vi "canDataSort.vi"() -> ()   [LabVIEW 2023] (continued)
\n       223  0CF102A7   00000004    8        30\t75\tE0\t2E\t80\tFF\tFF\tFD\r\n       247  1FFFFFFF   00000004    8        00\t00\tFF\tFF\tFF\tFF\tFF\tFF\r\n       246  18F121F0   00000004    8        09\t16\t00\t00\tFF\tFF\tB0\t01\r\n       246  18F106A7   00000004    8        00\tF7\tFF\tFF\tFF\tFF\tFF\t75\r\n       245  0CF104A7   00000004    8        F0\t60\t22\tFC\tFF\tFF\tFF\t3A\r\n       244  0CF103A7   00000004    8        17\t1F\t08\t60\tB1\t1F\t08\t3A\r\n       244  0CF102A7   00000004    8        30\t75\tE0\t2E\t80\tFF\tFF\tFD\r\n       243  0C3C4D4A   00000004    8        BE\tFF\tFF\t7F\t18\tFF\tFF\t3A\r\n       243  0CF101A7   00000004    8        68\t00\t97\tCC\t00\t15\t39\t26\r\n       242  18F120F0   00000004    8        2B\t75\t60\tB1\tB0\t01\tFF\tFF\r\n       241  18F11FF0   00000004    8        FF\t3F\t90\t68\t88\t1B\t10\tAC\r\n       232  1FFFFFFF   00000004    8        00\t00\tFF\tFF\tFF\tFF\tFF\tFF\r\n       252  1FFFFFFF   00000004    8        00\t00\tFF\tFF\tFF\tFF\tFF\tFF\r\n       247  1FFFFFFF   00000004    8        00\t00\tFF\tFF\tFF\tFF\tFF\tFF\r\n       246  18F121F0   00000004    8        09\t16\t00\t00\tFF\tFF\tB0\t01\r\n       246  18F106A7   00000004    8        00\tF7\tFF\tFF\tFF\tFF\tFF\t75\r\n       245  0CF104A7   00000004    8        F0\t60\t22\tFC\tFF\tFF\tFF\t3A\r\n       244  0CF103A7   00000004    8        17\t1F\t08\t60\tB1\t1F\t08\t3A\r\n       244  0CF102A7   00000004    8        30\t75\tE0\t2E\t80\tFF\tFF\tFD\r\n       243  0C3C4D4A   00000004    8        BE\tFF\tFF\t7F\t18\tFF\tFF\t3A\r\n       243  0CF101A7   00000004    8        68\t00\t97\tCC\t00\t15\t39\t26\r\n       242  18F120F0   00000004    8        2B\t75\t60\tB1\tB0\t01\tFF\tFF\r\n       241  18F11FF0   00000004    8        FF\t3F\t90\t68\t88\t1B\t10\tAC\r\n       262  1FFFFFFF   00000004    8        00\t20\tFF\tFF\tFF\tFF\tFF\tFF\r\n       252  1FFFFFFF   00000004    8        00\t00\tFF\tFF\tFF\tFF\tFF\tFF\r\n       247  1FFFFFFF   00000004    8        00\t00\tFF\tFF\tFF\tFF\tFF\tFF\r\n       246  18F121F0   00000004    8        09\t16\t00\t00\tFF\tFF\tB0\t01\r\n       246  18F106A7   00000004    8        00\tF7\tFF\tFF\tFF\tFF\tFF\t75\r\n       245  0CF104A7   00000004    8        F0\t60\t22\tFC\tFF\tFF\tFF\t3A\r\n       244  0CF103A7   00000004    8        17\t1F\t08\t60\tB1\t1F\t08\t3A\r\n       244  0CF102A7   00000004    8        30\t75\tE0\t2E\t80\tFF\tFF\tFD\r\n       243  0C3C4D4A   00000004    8        BE\tFF\tFF\t7F\t18\tFF\tFF\t3A\r\n       243  0CF101A7   00000004    8        68\t00\t97\tCC\t00\t15\t39\t26\r\n       242  18F120F0   00000004    8        2B\t75\t60\tB1\tB0\t01\tFF\tFF\r\n       263  0CF101A7   00000004    8        68\t00\t97\tCC\t00\t15\t39\t27\r\n       262  1FFFFFFF   00000004    8        00\t20\tFF\tFF\tFF\tFF\tFF\tFF\r\n       252  1FFFFFFF   00000004    8        00\t00\tFF\tFF\tFF\tFF\tFF\tFF\r\n       247  1FFFFFFF   00000004    8        00\t00\tFF\tFF\tFF\tFF\tFF\tFF\r\n       246  18F121F0   00000004    8        09\t16\t00\t00\tFF\tFF\tB0\t01\r\n       246  18F106A7   00000004    8        00\tF7\tFF\tFF\tFF\tFF\tFF\t75\r\n       245  0CF104A7   00000004    8        F0\t60\t22\tFC\tFF\tFF\tFF\t3A\r\n       244  0CF103A7   00000004    8        17\t1F\t08\t60\tB1\t1F\t08\t3A\r\n       244  0CF102A7   00000004    8        30\t75\tE0\t2E\t80\tFF\tFF\tFD\r\n       243  0C3C4D4A   00000004    8        BE\tFF\tFF\t7F\t18\tFF\tFF\t3A\r\n       243  0CF101A7   00000004    8        68\t00\t97\tCC\t00\t15\t39\t26\r\n       263  0CF102A7   00000004    8        30\t75\tE0\t2E\t80\tFF\tFF\tFD\r\n       263  0CF101A7   00000004    8        68\t00\t97\tCC\t00\t15\t39\t27\r\n       262  1FFFFFFF   00000004    8        00\t20\tFF\tFF\tFF\tFF\tFF\tFF\r\n       252  1FFFFFFF   00000004    8        00\t00\tFF\tFF\tFF\tFF\tFF\tFF\r\n       247  1FFFFFFF   00000004    8        00\t00\tFF\tFF\tFF\tFF\tFF\tFF\r\n       246  18F121F0   00000004    8        09\t16\t00\t00\tFF\tFF\tB0\t01\r\n       246  18F106A7   00000004    8        00\tF7\tFF\tFF\tFF\tFF\tFF\t75\r\n       245  0CF104A7   00000004    8        F0\t60\t22\tFC\tFF\tFF\tFF\t3A\r\n       244  0CF103A7   00000004    8        17\t1F\t08\t60\tB1\t1F\t08\t3A\r\n       244  0CF102A7   00000004    8        30\t75\tE0\t2E\t80\tFF\tFF\tFD\r\n       243  0C3C4D4A   00000004    8        BE\tFF\tFF\t7F\t18\tFF\tFF\t3A\r\n       272  1FFFFFFF   00000004    8        00\t00\tFF\tFF\tFF\tFF\tFF\tFF\r\n       263  0CF102A7   00000004    8        30\t75\tE0\t2E\t80\tFF\tFF\tFD\r\n       263  0CF101A7   00000004    8        68\t00\t97\tCC\t00\t15\t39\t27\r\n       262  1FFFFFFF   00000004    8        00\t20\tFF\tFF\tFF\tFF\tFF\tFF\r\n       252  1FFFFFFF   00000004    8        00\t00\tFF\tFF\tFF\tFF\tFF\tFF\r\n       247  1FFFFFFF   00000004    8        00\t00\tFF\tFF\tFF\tFF\tFF\tFF\r\n       246  18F121F0   00000004    8        09\t16\t00\t00\tFF\tFF\tB0\t01\r\n       246  18F106A7   00000004    8        00\tF7\tFF\tFF\tFF\tFF\tFF\t75\r\n       245  0CF104A7   00000004    8        F0\t60\t22\tFC\tFF\tFF\tFF\t3A\r\n       244  0CF103A7   00000004    8        17\t1F\t08\t60\tB1\t1F\t08\t3A\r\n       244  0CF102A7   00000004    8        30\t75\tE0\t2E\t80\tFF\tFF\tFD\r\n       282  1FFFFFFF   00000004    8        00\t00\tFF\tFF\tFF\tFF\tFF\tFF\r\n       272  1FFFFFFF   00000004    8        00\t00\tFF\tFF\tFF\tFF\tFF\tFF\r\n       263  0CF102A7   00000004    8        30\t75\tE0\t2E\t80\tFF\tFF\tFD\r\n       263  0CF101A7   00000004    8        68\t00\t97\tCC\t00\t15\t39\t27\r\n       262  1FFFFFFF   00000004    8        00\t20\tFF\tFF\tFF\tFF\tFF\tFF\r\n       252  1FFFFFFF   00000004    8        00\t00\tFF\tFF\tFF\tFF\tFF\tFF\r\n       247  1FFFFFFF   00000004    8        00\t00\tFF\tFF\tFF\tFF\tFF\tFF\r\n       246  18F121F0   00000004    8        09\t16\t00\t00\tFF\tFF\tB0\t01\r\n       246  18F106A7   00000004    8        00\tF7\tFF\tFF\tFF\tFF\tFF\t75\r\n       245  0CF104A7   00000004    8        F0\t60\t22\tFC\tFF\tFF\tFF\t3A\r\n       244  0CF103A7   00000004    8        17\t1F\t08\t60\tB1\t1F\t08\t3A\r\n       283  0CF101A7   00000004    8        68\t00\t97\tCC\t00\t15\t39\t28\r\n       282  1FFFFFFF   00000004    8        00\t00\tFF\tFF\tFF\tFF\tFF\tFF\r\n       272  1FFFFFFF   00000004    8        00\t00\tFF\tFF\tFF\tFF\tFF\tFF\r\n       263  0CF102A7   00000004    8        30\t75\tE0\t2E\t80\tFF\tFF\tFD\r\n       263  0CF101A7   00000004    8        68\t00\t97\tCC\t00\t15\t39\t27\r\n       262  1FFFFFFF   00000004    8        00\t20\tFF\tFF\tFF\tFF\tFF\tFF\r\n       252  1FFFFFFF   00000004    8        00\t00\tFF\tFF\tFF\tFF\tFF\tFF\r\n       247  1FFFFFFF   00000004    8        00\t00\tFF\tFF\tFF\tFF\tFF\tFF\r\n       246  18F121F0   00000004    8        09\t16\t00\t00\tFF\tFF\tB0\t01\r\n       246  18F106A7   00000004    8        00\tF7\tFF\tFF\tFF\tFF\tFF\t75\r\n       245  0CF104A7   00000004    8        F0\t60\t22\tFC\tFF\tFF\tFF\t3A\r\n       283  0CF102A7   00000004    8        30\t75\tE0\t2E\t80\tFF\tFF\tFD\r\n       283  0CF101A7   00000004    8        68\t00\t97\tCC\t00\t15\t39\t28\r\n       282  1FFFFFFF   00000004    8        00\t00\tFF\tFF\tFF\tFF\tFF\tFF\r\n       272  1FFFFFFF   00000004    8        00\t00\tFF\tFF\tFF\tFF\tFF\tFF\r\n       263  0CF102A7   00000004    8        30\t75\tE0\t2E\t80\tFF\tFF\tFD\r\n       263  0CF101A7   00000004    8        68\t00\t97\tCC\t00\t15\t39\t27\r\n       262  1FFFFFFF   00000004    8        00\t20\tFF\tFF\tFF\tFF\tFF\tFF\r\n       252  1FFFFFFF   00000004    8        00\t00\tFF\tFF\tFF\tFF\tFF\tFF\r\n       247  1FFFFFFF   00000004    8        00\t00\tFF\tFF\tFF\tFF\tFF\tFF\r\n       246  18F121F0   00000004    8        09\t16\t00\t00\tFF\tFF\tB0\t01\r\n       246  18F106A7   00000004    8        00\tF7\tFF\tFF\tFF\tFF\tFF\t75\r\n       292  1FFFFFFF   00000004    8        00\t00\tFF\tFF\tFF\tFF\tFF\tFF\r\n       283  0CF102A7   00000004    8        30\t75\tE0\t2E\t80\tFF\tFF\tFD\r\n       283  0CF101A7   00000004    8        68\t00\t97\tCC\t00\t15\t39\t28\r\n       282  1FFFFFFF   00000004    8        00\t00\tFF\tFF\tFF\tFF\tFF\tFF\r\n       272  1FFFFFFF   00000004    8        00\t00\tFF\tFF\tFF\tFF\tFF\tFF\r\n       263  0CF102A7   00000004    8        30\t75\tE0\t2E\t80\tFF\tFF\tFD\r\n       263  0CF101A7   00000004    8        68\t00\t97\tCC\t00\t15\t39\t27\r\n       262  1FFFFFFF   00000004    8        00\t20\tFF\tFF\tFF\tFF\tFF\tFF\r\n       252  1FFFFFFF   00000004    8        00\t00\tFF\tFF\tFF\tFF\tFF\tFF\r\n       247  1FFFFFFF   00000004    8        00\t00\tFF\tFF\tFF\tFF\tFF\tFF\r\n       246  18F121F0   00000004    8        09\t16\t00\t00\tFF\tFF\tB0\t01\r\n       293  18F106A7   00000004    8        00\tF7\tFF\tFF\tFF\tFF\tFF\t76\r\n       292  1FFFFFFF   00000004    8        00\t00\tFF\tFF\tFF\tFF\tFF\tFF\r\n       283  0CF102A7   00000004    8        30\t75\tE0\t2E\t80\tFF\tFF\tFD\r\n       283  0CF101A7   00000004    8        68\t00\t97\tCC\t00\t15\t39\t28\r\n       282  1FFFFFFF   00000004    8        00\t00\tFF\tFF\tFF\tFF\tFF\tFF\r\n       272  1FFFFFFF   00000004    8        00\t00\tFF\tFF\tFF\tFF\tFF\tFF\r\n       263  0CF102A7   00000004    8        30\t75\tE0\t2E\t80\tFF\tFF\tFD\r\n       263  0CF101A7   00000004    8        68\t00\t97\tCC\t00\t15\t39\t27\r\n       262  1FFFFFFF   00000004    8        00\t20\tFF\tFF\tFF\tFF\tFF\tFF\r\n       252  1FFFFFFF   00000004    8        00\t00\tFF\tFF\tFF\tFF\tFF\tFF\r\n       247  1FFFFFFF   00000004    8        00\t00\tFF\tFF\tFF\tFF\tFF\tFF\r\n       302  1FFFFFFF   00000004    8        00\t00\tFF\tFF\tFF\tFF\tFF\tFF\r\n       293  18F106A7   00000004    8        00\tF7\tFF\tFF\tFF\tFF\tFF\t76\r\n       292  1FFFFFFF   00000004    8        00\t00\tFF\tFF\tFF\tFF\tFF\tFF\r\n       283  0CF102A7   00000004    8        30\t75\tE0\t2E\t80\tFF\tFF\tFD\r\n       283  0CF101A7   00000004    8        68\t00\t97\tCC\t00\t15\t39\t28\r\n       282  1FFFFFFF   00000004    8        00\t00\tFF\tFF\tFF\tFF\tFF\tFF\r\n       272  1FFFFFFF   00000004    8        00\t00\tFF\tFF\tFF\tFF\tFF\tFF\r\n       263  0CF102A7   00000004    8        30\t75\tE0\t2E\t80\tFF\tFF\tFD\r\n       263  0CF101A7   00000004    8        68\t00\t97\tCC\t00\t15\t39\t27\r\n       262  1FFFFFFF   00000004    8        00\t20\tFF\tFF\tFF\tFF\tFF\tFF\r\n       252  1FFFFFFF   00000004    8        00\t00\tFF\tFF\tFF\tFF\tFF\tFF\r\n       303  0CF101A7   00000004    8        68\t00\t97\tCC\t00\t15\t39\t29\r\n       302  1FFFFFFF   00000004    8        00\t00\tFF\tFF\tFF\tFF\tFF\tFF\r\n       293  18F106A7   00000004    8        00\tF7\tFF\tFF\tFF\tFF\tFF\t76\r\n       292  1FFFFFFF   00000004    8        00\t00\tFF\tFF\tFF\tFF\tFF\tFF\r\n       283  0CF102A7   00000004    8        30\t75\tE0\t2E\t80\tFF\tFF\tFD\r\n       283  0CF101A7   00000004    8        68\t00\t97\tCC\t00\t15\t39\t28\r\n       282  1FFFFFFF   00000004    8        00\t00\tFF\tFF\tFF\tFF\tFF\tFF\r\n       272  1FFFFFFF   00000004    8        00\t00\tFF\tFF\tFF\tFF\tFF\tFF\r\n       263  0CF102A7   00000004    8        30\t75\tE0\t2E\t80\tFF\tFF\tFD\r\n       263  0CF101A7   00000004    8        68\t00\t97\tCC\t00\t15\t39\t27\r\n       262  1FFFFFFF   00000004    8        00\t20\tFF\tFF\tFF\tFF\tFF\tFF\r\n       303  0CF102A7   00000004    8        30\t75\tE0\t2E\t80\tFF\tFF\tFD\r\n       303  0CF101A7   00000004    8        68\t00\t97\tCC\t00\t15\t39\t29\r\n       302  1FFFFFFF   00000004    8        00\t00\tFF\tFF\tFF\tFF\tFF\tFF\r\n       293  18F106A7   00000004    8        00\tF7\tFF\tFF\tFF\tFF\tFF\t76\r\n       292  1FFFFFFF   00000004    8        00\t00\tFF\tFF\tFF\tFF\tFF\tFF\r\n       283  0CF102A7   00000004    8        30\t75\tE0\t2E\t80\tFF\tFF\tFD\r\n       283  0CF101A7   00000004    8        68\t00\t97\tCC\t00\t15\t39\t28\r\n       282  1FFFFFFF   00000004    8        00\t00\tFF\tFF\tFF\tFF\tFF\tFF\r\n       272  1FFFFFFF   00000004    8        00\t00\tFF\tFF\tFF\tFF\tFF\tFF\r\n       263  0CF102A7   00000004    8        30\t75\tE0\t2E\t80\tFF\tFF\tFD\r\n       263  0CF101A7   00000004    8        68\t00\t97\tCC\t00\t15\t39\t27\r\n       312  1FFFFFFF   00000004    8        00\t20\tFF\tFF\tFF\tFF\tFF\tFF\r\n       303  0CF102A7   00000004    8        30\t75\tE0\t2E\t80\tFF\tFF\tFD\r\n       303  0CF101A7   00000004    8        68\t00\t97\tCC\t00\t15\t39\t29\r\n       302  1FFFFFFF   00000004    8        00\t00\tFF\tFF\tFF\tFF\tFF\tFF\r\n       293  18F106A7   00000004    8        00\tF7\tFF\tFF\tFF\tFF\tFF\t76\r\n       292  1FFFFFFF   00000004    8        00\t00\tFF\tFF\tFF\tFF\tFF\tFF\r\n       283  0CF102A7   00000004    8        30\t75\tE0\t2E\t80\tFF\tFF\tFD\r\n       283  0CF101A7   00000004    8        68\t00\t97\tCC\t00\t15\t39\t28\r\n       282  1FFFFFFF   00000004    8        00\t00\tFF\tFF\tFF\tFF\tFF\tFF\r\n       272  1FFFFFFF   00000004    8        00\t00\tFF\tFF\tFF\tFF\tFF\tFF\r\n       263  0CF102A7   00000004    8        30\t75\tE0\t2E\t80\tFF\tFF\tFD\r\n       322  1FFFFFFF   00000004    8        00\t20\tFF\tFF\tFF\tFF\tFF\tFF\r\n       312  1FFFFFFF   00000004    8        00\t20\tFF\tFF\tFF\tFF\tFF\tFF\r\n       303  0CF102A7   00000004    8        30\t75\tE0\t2E\t80\tFF\tFF\tFD\r\n       303  0CF101A7   00000004    8        68\t00\t97\tCC\t00\t15\t39\t29\r\n       302  1FFFFFFF   00000004    8        00\t00\tFF\tFF\tFF\tFF\tFF\tFF\r\n       293  18F106A7   00000004    8        00\tF7\tFF\tFF\tFF\tFF\tFF\t76\r\n       292  1FFFFFFF   00000004    8        00\t00\tFF\tFF\tFF\tFF\tFF\tFF\r\n       283  0CF102A7   00000004    8        30\t75\tE0\t2E\t80\tFF\tFF\tFD\r\n       283  0CF101A7   00000004    8        68\t00\t97\tCC\t00\t15\t39\t28\r\n       282  1FFFFFFF   00000004    8        00\t00\tFF\tFF\tFF\tFF\tFF\tFF\r\n       272  1FFFFFFF   00000004    8        00\t00\tFF\tFF\tFF\tFF\tFF\tFF\r\n       323  0CF101A7   00000004    8        68\t00\t97\tCC\t00\t15\t39\t2A\r\n       322  1FFFFFFF   00000004    8        00\t20\tFF\tFF\tFF\tFF\tFF\tFF\r\n       312  1FFFFFFF   00000004    8        00\t20\tFF\tFF\tFF\tFF\tFF\tFF\r\n       303  0CF102A7   00000004    8        30\t75\tE0\t2E\t80\tFF\tFF\tFD\r\n       303  0CF101A7   00000004    8        68\t00\t97\tCC\t00\t15\t39\t29\r\n       302  1FFFFFFF   00000004    8        00\t00\tFF\tFF\tFF\tFF\tFF\tFF\r\n       293  18F106A7   00000004    8        00\tF7\tFF\tFF\tFF\tFF\tFF\t76\r\n       292  1FFFFFFF   00000004    8        00\t00\tFF\tFF\tFF\tFF\tFF\tFF\r\n       283  0CF102A7   00000004    8        30\t75\tE0\t2E\t80\tFF\tFF\tFD\r\n       283  0CF101A7   00000004    8        68\t00\t97\tCC\t00\t15\t39\t28\r\n       282  1FFFFFFF   00000004    8        00\t00\tFF\tFF\tFF\tFF\tFF\tFF\r\n       323  0CF102A7   00000004    8        30\t75\tE0\t2E\t80\tFF\tFF\tFD\r\n       323  0CF101A7   00000004    8        68\t00\t97\tCC\t00\t15\t39\t2A\r\n       322  1FFFFFFF   00000004    8        00\t20\tFF\tFF\tFF\tFF\tFF\tFF\r\n       312  1FFFFFFF   00000004    8        00\t20\tFF\tFF\tFF\tFF\tFF\tFF\r\n       303  0CF102A7   00000004    8        30\t75\tE0\t2E\t80\tFF\tFF\tFD\r\n       303  0CF101A7   00000004    8        68\t00\t97\tCC\t00\t15\t39\t29\r\n       302  1FFFFFFF   00000004    8        00\t00\tFF\tFF\tFF\tFF\tFF\tFF\r\n       293  18F106A7   00000004    8        00\tF7\tFF\tFF\tFF\tFF\tFF\t76\r\n       292  1FFFFFFF   00000004    8        00\t00\tFF\tFF\tFF\tFF\tFF\tFF\r\n       283  0CF102A7   00000004    8        30\t75\tE0\t2E\t80\tFF\tFF\tFD\r\n       283  0CF101A7   00000004    8        68\t00\t97\tCC\t00\t15\t39\t28\r\n       332  1FFFFFFF   00000004    8        00\t00\tFF\tFF\tFF\tFF\tFF\tFF\r\n       323  0CF102A7   00000004    8        30\t75\tE0\t2E\t80\tFF\tFF\tFD\r\n       323  0CF101A7   00000004    8        68\t00\t97\tCC\t00\t15\t39\t2A\r\n       322  1FFFFFFF   00000004    8        00\t20\tFF\tFF\tFF\tFF\tFF\tFF\r\n       312  1FFFFFFF   00000004    8        00\t20\tFF\tFF\tFF\tFF\tFF\tFF\r\n       303  0CF102A7   00000004    8        30\t75\tE0\t2E\t80\tFF\tFF\tFD\r\n       303  0CF101A7   00000004    8        68\t00\t97\tCC\t00\t15\t39\t29\r\n       302  1FFFFFFF   00000004    8        00\t00\tFF\tFF\tFF\tFF\tFF\tFF\r\n       293  18F106A7   00000004    8        00\tF7\tFF\tFF\tFF\tFF\tFF\t76\r\n       292  1FFFFFFF   00000004    8        00\t00\tFF\tFF\tFF\tFF\tFF\tFF\r\n       283  0CF102A7   00000004    8        30\t75\tE0\t2E\t80\tFF\tFF\tFD\r\n       341  18F11FF0   00000004    8        FF\t3F\t90\t68\t88\t1B\t10\tBC\r\n       332  1FFFFFFF   00000004    8        00\t00\tFF\tFF\tFF\tFF\tFF\tFF\r\n       323  0CF102A7   00000004    8        30\t75\tE0\t2E\t80\tFF\tFF\tFD\r\n       323  0CF101A7   00000004    8        68\t00\t97\tCC\t00\t15\t39\t2A\r\n       322  1FFFFFFF   00000004    8        00\t20\tFF\tFF\tFF\tFF\tFF\tFF\r\n       312  1FFFFFFF   00000004    8        00\t20\tFF\tFF\tFF\tFF\tFF\tFF\r\n       303  0CF102A7   00000004    8        30\t75\tE0\t2E\t80\tFF\tFF\tFD\r\n       303  0CF101A7   00000004    8        68\t00\t97\tCC\t00\t15\t39\t29\r\n       302  1FFFFFFF   00000004    8        00\t00\tFF\tFF\tFF\tFF\tFF\tFF\r\n       293  18F106A7   00000004    8        00\tF7\tFF\tFF\tFF\tFF\tFF\t76\r\n       292  1FFFFFFF   00000004    8        00\t00\tFF\tFF\tFF\tFF\tFF\tFF\r\n       342  18F120F0   00000004    8        2B\t75\t60\tB1\tB0\t01\tFF\tFF\r\n       341  18F11FF0   00000004    8        FF\t3F\t90\t68\t88\t1B\t10\tBC\r\n       332  1FFFFFFF   00000004    8        00\t00\tFF\tFF\tFF\tFF\tFF\tFF\r\n       323  0CF102A7   00000004    8        30\t75\tE0\t2E\t80\tFF\tFF\tFD\r\n       323  0CF101A7   00000004    8        68\t00\t97\tCC\t00\t15\t39\t2A\r\n       322  1FFFFFFF   00000004    8        00\t20\tFF\tFF\tFF\tFF\tFF\tFF\r\n       312  1FFFFFFF   00000004    8        00\t20\tFF\tFF\tFF\tFF\tFF\tFF\r\n       303  0CF102A7   00000004    8        30\t75\tE0\t2E\t80\tFF\tFF\tFD\r\n       303  0CF101A7   00000004    8        68\t00\t97\tCC\t00\t15\t39\t29\r\n       302  1FFFFFFF   00000004    8        00\t00\tFF\tFF\tFF\tFF\tFF\tFF\r\n       293  18F106A7   00000004    8        00\tF7\tFF\tFF\tFF\tFF\tFF\t76\r\n       343  0CF101A7   00000004    8        68\t00\t97\tCC\t00\t15\t39\t2B\r\n       342  18F120F0   00000004    8        2B\t75\t60\tB1\tB0\t01\tFF\tFF\r\n       341  18F11FF0   00000004    8        FF\t3F\t90\t68\t88\t1B\t10\tBC\r\n       332  1FFFFFFF   00000004    8        00\t00\tFF\tFF\tFF\tFF\tFF\tFF\r\n       323  0CF102A7   00000004    8        30\t75\tE0\t2E\t80\tFF\tFF\tFD\r\n       323  0CF101A7   00000004    8        68\t00\t97\tCC\t00\t15\t39\t2A\r\n       322  1FFFFFFF   00000004    8        00\t20\tFF\tFF\tFF\tFF\tFF\tFF\r\n       312  1FFFFFFF   00000004    8        00\t20\tFF\tFF\tFF\tFF\tFF\tFF\r\n       303  0CF102A7   00000004    8        30\t75\tE0\t2E\t80\tFF\tFF\tFD\r\n       303  0CF101A7   00000004    8        68\t00\t97\tCC\t00\t15\t39\t29\r\n       302  1FFFFFFF   00000004    8        00\t00\tFF\tFF\tFF\tFF\tFF\tFF\r\n       343  0C3C4D4A   00000004    8        BE\tFF\tFF\t7F\t18\tFF\tFF\t3B\r\n       343  0CF101A7   00000004    8        68\t00\t97\tCC\t00\t15\t39\t2B\r\n       342  18F120F0   00000004    8        2B\t75\t60\tB1\tB0\t01\tFF\tFF\r\n       341  18F11FF0   00000004    8        FF\t3F\t90\t68\t88\t1B\t10\tBC\r\n       332  1FFFFFFF   00000004    8        00\t00\tFF\tFF\tFF\tFF\tFF\tFF\r\n       323  0CF102A7   00000004    8        30\t75\tE0\t2E\t80\tFF\tFF\tFD\r\n       323  0CF101A7   00000004    8        68\t00\t97\tCC\t00\t15\t39\t2A\r\n       322  1FFFFFFF   00000004    8        00\t20\tFF\tFF\tFF\tFF\tFF\tFF\r\n       312  1FFFFFFF   00000004    8        00\t20\tFF\tFF\tFF\tFF\tFF\tFF\r\n       303  0CF102A7   00000004    8        30\t75\tE0\t2E\t80\tFF\tFF\tFD\r\n       303  0CF101A7   00000004    8        68\t00\t97\tCC\t00\t15\t39\t29\r\n       344  0CF102A7   00000004    8        30\t75\tE0\t2E\t80\tFF\tFF\tFD\r\n       343  0C3C4D4A   00000004    8        BE\tFF\tFF\t7F\t18\tFF\tFF\t3B\r\n       343  0CF101A7   00000004    8        68\t00\t97\tCC\t00\t15\t39\t2B\r\n       342  18F120F0   00000004    8        2B\t75\t60\tB1\tB0\t01\tFF\tFF\r\n       341  18F11FF0   00000004    8        FF\t3F\t90\t68\t88\t1B\t10\tBC\r\n       332  1FFFFFFF   00000004    8        00\t00\tFF\tFF\tFF\tFF\tFF\tFF\r\n       323  0CF102A7   00000004    8        30\t75\tE0\t2E\t80\tFF\tFF\tFD\r\n       323  0CF101A7   00000004    8        68\t00\t97\tCC\t00\t15\t39\t2A\r\n       322  1FFFFFFF   00000004    8        00\t20\tFF\tFF\tFF\tFF\tFF\tFF\r\n       312  1FFFFFFF   00000004    8        00\t20\tFF\tFF\tFF\tFF\tFF\tFF\r\n       303  0CF102A7   00000004    8        30\t75\tE0\t2E\t80\tFF\tFF\tFD\r\n       344  0CF103A7   00000004    8        17\t1F\t08\t60\tB1\t1F\t08\t3B\r\n       344  0CF102A7   00000004    8        30\t75\tE0\t2E\t80\tFF\tFF\tFD\r\n       343  0C3C4D4A   00000004    8        BE\tFF\tFF\t7F\t18\tFF\tFF\t3B\r\n       343  0CF101A7   00000004    8        68\t00\t97\tCC\t00\t15\t39\t2B\r\n       342  18F120F0   00000004    8        2B\t75\t60\tB1\tB0\t01\tFF\tFF\r\n       341  18F11FF0   00000004    8        FF\t3F\t90\t68\t88\t1B\t10\tBC\r\n       332  1FFFFFFF   00000004    8        00\t00\tFF\tFF\tFF\tFF\tFF\tFF\r\n       323  0CF102A7   00000004    8        30\t75\tE0\t2E\t80\tFF\tFF\tFD\r\n       323  0CF101A7   00000004    8        68\t00\t97\tCC\t00\t15\t39\t2A\r\n       322  1FFFFFFF   00000004    8        00\t20\tFF\tFF\tFF\tFF\tFF\tFF\r\n       312  1FFFFFFF   00000004    8        00\t20\tFF\tFF\tFF\tFF\tFF\tFF\r\n       345  0CF104A7   00000004    8        F0\t60\t22\tFC\tFF\tFF\tFF\t3B\r\n       344  0CF103A7   00000004    8        17\t1F\t08\t60\tB1\t1F\t08\t3B\r\n       344  0CF102A7   00000004    8        30\t75\tE0\t2E\t80\tFF\tFF\tFD\r\n       343  0C3C4D4A   00000004    8        BE\tFF\tFF\t7F\t18\tFF\tFF\t3B\r\n       343  0CF101A7   00000004    8        68\t00\t97\tCC\t00\t15\t39\t2B\r\n       342  18F120F0   00000004    8        2B\t75\t60\tB1\tB0\t01\tFF\tFF\r\n       341  18F11FF0   00000004    8        FF\t3F\t90\t68\t88\t1B\t10\tBC\r\n       332  1FFFFFFF   00000004    8        00\t00\tFF\tFF\tFF\tFF\tFF\tFF\r\n       323  0CF102A7   00000004    8        30\t75\tE0\t2E\t80\tFF\tFF\tFD\r\n       323  0CF101A7   00000004    8        68\t00\t97\tCC\t00\t15\t39\t2A\r\n       322  1FFFFFFF   00000004    8        00\t20\tFF\tFF\tFF\tFF\tFF\tFF\r\n       345  18F106A7   00000004    8        00\tF7\tFF\tFF\tFF\tFF\tFF\t77\r\n       345  0CF104A7   00000004    8        F0\t60\t22\tFC\tFF\tFF\tFF\t3B\r\n       344  0CF103A7   00000004    8        17\t1F\t08\t60\tB1\t1F\t08\t3B\r\n       344  0CF102A7   00000004    8        30\t75\tE0\t2E\t80\tFF\tFF\tFD\r\n       343  0C3C4D4A   00000004    8        BE\tFF\tFF\t7F\t18\tFF\tFF\t3B\r\n       343  0CF101A7   00000004    8        68\t00\t97\tCC\t00\t15\t39\t2B\r\n       342  18F120F0   00000004    8        2B\t75\t60\tB1\tB0\t01\tFF\tFF\r\n       341  18F11FF0   00000004    8        FF\t3F\t90\t68\t88\t1B\t10\tBC\r\n       332  1FFFFFFF   00000004    8        00\t00\tFF\tFF\tFF\tFF\tFF\tFF\r\n       323  0CF102A7   00000004    8        30\t75\tE0\t2E\t80\tFF\tFF\tFD\r\n       323  0CF101A7   00000004    8        68\t00\t97\tCC\t00\t15\t39\t2A\r\n       346  18F121F0   00000004    8        09\t16\t00\t00\tFF\tFF\tB0\t01\r\n       345  18F106A7   00000004    8        00\tF7\tFF\tFF\tFF\tFF\tFF\t77\r\n       345  0CF104A7   00000004    8        F0\t60\t22\tFC\tFF\tFF\tFF\t3B\r\n       344  0CF103A7   00000004    8        17\t1F\t08\t60\tB1\t1F\t08\t3B\r\n       344  0CF102A7   00000004    8        30\t75\tE0\t2E\t80\tFF\tFF\tFD\r\n       343  0C3C4D4A   00000004    8        BE\tFF\tFF\t7F\t18\tFF\tFF\t3B\r\n       343  0CF101A7   00000004    8        68\t00\t97\tCC\t00\t15\t39\t2B\r\n       342  18F120F0   00000004    8        2B\t75\t60\tB1\tB0\t01\tFF\tFF\r\n       341  18F11FF0   00000004    8        FF\t3F\t90\t68\t88\t1B\t10\tBC\r\n       332  1FFFFFFF   00000004    8        00\t00\tFF\tFF\tFF\tFF\tFF\tFF\r\n       323  0CF102A7   00000004    8        30\t75\tE0\t2E\t80\tFF\tFF\tFD\r\n       347  1FFFFFFF   00000004    8        00\t00\tFF\tFF\tFF\tFF\tFF\tFF\r\n       346  18F121F0   00000004    8        09\t16\t00\t00\tFF\tFF\tB0\t01\r\n       345  18F106A7   00000004    8        00\tF7\tFF\tFF\tFF\tFF\tFF\t77\r\n       345  0CF104A7   00000004    8        F0\t60\t22\tFC\tFF\tFF\tFF\t3B\r\n       344  0CF103A7   00000004    8        17\t1F\t08\t60\tB1\t1F\t08\t3B\r\n       344  0CF102A7   00000004    8        30\t75\tE0\t2E\t80\tFF\tFF\tFD\r\n       343  0C3C4D4A   00000004    8        BE\tFF\tFF\t7F\t18\tFF\tFF\t3B\r\n       343  0CF101A7   00000004    8        68\t00\t97\tCC\t00\t15\t39\t2B\r\n       342  18F120F0   00000004    8        2B\t75\t60\tB1\tB0\t01\tFF\tFF\r\n       341  18F11FF0   00000004    8        FF\t3F\t90\t68\t88\t1B\t10\tBC\r\n       332  1FFFFFFF   00000004    8        00\t00\tFF\tFF\tFF\tFF\tFF\tFF\r\n       352  1FFFFFFF   00000004    8        00\t00\tFF\tFF\tFF\tFF\tFF\tFF\r\n       347  1FFFFFFF   00000004    8        00\t00\tFF\tFF\tFF\tFF\tFF\tFF\r\n       346  18F121F0   00000004    8        09\t16\t00\t00\tFF\tFF\tB0\t01\r\n       345  18F106A7   00000004    8        00\tF7\tFF\tFF\tFF\tFF\tFF\t77\r\n       345  0CF104A7   00000004    8        F0\t60\t22\tFC\tFF\tFF\tFF\t3B\r\n       344  0CF103A7   00000004    8        17\t1F\t08\t60\tB1\t1F\t08\t3B\r\n       344  0CF102A7   00000004    8        30\t75\tE0\t2E\t80\tFF\tFF\tFD\r\n       343  0C3C4D4A   00000004    8        BE\tFF\tFF\t7F\t18\tFF\tFF\t3B\r\n       343  0CF101A7   00000004    8        68\t00\t97\tCC\t00\t15\t39\t2B\r\n       342  18F120F0   00000004    8        2B\t75\t60\tB1\tB0\t01\tFF\tFF\r\n       341  18F11FF0   00000004    8        FF\t3F\t90\t68\t88\t1B\t10\tBC\r\n       362  1FFFFFFF   00000004    8        00\t00\tFF\tFF\tFF\tFF\tFF\tFF\r\n       352  1FFFFFFF   00000004    8        00\t00\tFF\tFF\tFF\tFF\tFF\tFF\r\n       347  1FFFFFFF   00000004    8        00\t00\tFF\tFF\tFF\tFF\tFF\tFF\r\n       346  18F121F0   00000004    8        09\t16\t00\t00\tFF\tFF\tB0\t01\r\n       345  18F106A7   00000004    8        00\tF7\tFF\tFF\tFF\tFF\tFF\t77\r\n       345  0CF104A7   00000004    8        F0\t60\t22\tFC\tFF\tFF\tFF\t3B\r\n       344  0CF103A7   00000004    8        17\t1F\t08\t60\tB1\t1F\t08\t3B\r\n       344  0CF102A7   00000004    8        30\t75\tE0\t2E\t80\tFF\tFF\tFD\r\n       343  0C3C4D4A   00000004    8        BE\tFF\tFF\t7F\t18\tFF\tFF\t3B\r\n       343  0CF101A7   00000004    8        68\t00\t97\tCC\t00\t15\t39\t2B\r\n       342  18F120F0   00000004    8        2B\t75\t60\tB1\tB0\t01\tFF\tFF\r\n       363  0CF101A7   00000004    8        68\t00\t97\tCC\t00\t15\t39\t2C\r\n       362  1FFFFFFF   00000004    8        00\t00\tFF\tFF\tFF\tFF\tFF\tFF\r\n       352  1FFFFFFF   00000004    8        00\t00\tFF\tFF\tFF\tFF\tFF\tFF\r\n       347  1FFFFFFF   00000004    8        00\t00\tFF\tFF\tFF\tFF\tFF\tFF\r\n       346  18F121F0   00000004    8        09\t16\t00\t00\tFF\tFF\tB0\t01\r\n       345  18F106A7   00000004    8        00\tF7\tFF\tFF\tFF\tFF\tFF\t77\r\n       345  0CF104A7   00000004    8        F0\t60\t22\tFC\tFF\tFF\tFF\t3B\r\n       344  0CF103A7   00000004    8        17\t1F\t08\t60\tB1\t1F\t08\t3B\r\n       344  0CF102A7   00000004    8        30\t75\tE0\t2E\t80\tFF\tFF\tFD\r\n       343  0C3C4D4A   00000004    8        BE\tFF\tFF\t7F\t18\tFF\tFF\t3B\r\n       343  0CF101A7   00000004    8        68\t00\t97\tCC\t00\t15\t39\t2B\r\n       363  0CF102A7   00000004    8        30\t75\tE0\t2E\t80\tFF\tFF\tFD\r\n       363  0CF101A7   00000004    8        68\t00\t97\tCC\t00\t15\t39\t2C\r\n       362  1FFFFFFF   00000004    8        00\t00\tFF\tFF\tFF\tFF\tFF\tFF\r\n       352  1FFFFFFF   00000004    8        00\t00\tFF\tFF\tFF\tFF\tFF\tFF\r\n       347  1FFFFFFF   00000004    8        00\t00\tFF\tFF\tFF\tFF\tFF\tFF\r\n       346  18F121F0   00000004    8        09\t16\t00\t00\tFF\tFF\tB0\t01\r\n       345  18F106A7   00000004    8        00\tF7\tFF\tFF\tFF\tFF\tFF\t77\r\n       345  0CF104A7   00000004    8        F0\t60\t22\tFC\tFF\tFF\tFF\t3B\r\n       344  0CF103A7   00000004    8        17\t1F\t08\t60\tB1\t1F\t08\t3B\r\n       344  0CF102A7   00000004    8        30\t75\tE0\t2E\t80\tFF\tFF\tFD\r\n       343  0C3C4D4A   00000004    8        BE\tFF\tFF\t7F\t18\tFF\tFF\t3B\r\n       372  1FFFFFFF   00000004    8        00\t20\tFF\tFF\tFF\tFF\tFF\tFF\r\n       363  0CF102A7   00000004    8        30\t75\tE0\t2E\t80\tFF\tFF\tFD\r\n       363  0CF101A7   00000004    8        68\t00\t97\tCC\t00\t15\t39\t2C\r\n       362  1FFFFFFF   00000004    8        00\t00\tFF\tFF\tFF\tFF\tFF\tFF\r\n       352  1FFFFFFF   00000004    8        00\t00\tFF\tFF\tFF\tFF\tFF\tFF\r\n       347  1FFFFFFF   00000004    8        00\t00\tFF\tFF\tFF\tFF\tFF\tFF\r\n       346  18F121F0   00000004    8        09\t16\t00\t00\tFF\tFF\tB0\t01\r\n       345  18F106A7   00000004    8        00\tF7\tFF\tFF\tFF\tFF\tFF\t77\r\n       345  0CF104A7   00000004    8        F0\t60\t22\tFC\tFF\tFF\tFF\t3B\r\n       344  0CF103A7   00000004    8        17\t1F\t08\t60\tB1\t1F\t08\t3B\r\n       344  0CF102A7   00000004    8        30\t75\tE0\t2E\t80\tFF\tFF\tFD\r\n       382  1FFFFFFF   00000004    8        00\t00\tFF\tFF\tFF\tFF\tFF\tFF\r\n       372  1FFFFFFF   00000004    8        00\t20\tFF\tFF\tFF\tFF\tFF\tFF\r\n       363  0CF102A7   00000004    8        30\t75\tE0\t2E\t80\tFF\tFF\tFD\r\n       363  0CF101A7   00000004    8        68\t00\t97\tCC\t00\t15\t39\t2C\r\n       362  1FFFFFFF   00000004    8        00\t00\tFF\tFF\tFF\tFF\tFF\tFF\r\n       352  1FFFFFFF   00000004    8        00\t00\tFF\tFF\tFF\tFF\tFF\tFF\r\n       347  1FFFFFFF   00000004    8        00\t00\tFF\tFF\tFF\tFF\tFF\tFF\r\n       346  18F121F0   00000004    8        09\t16\t00\t00\tFF\tFF\tB0\t01\r\n       345  18F106A7   00000004    8        00\tF7\tFF\tFF\tFF\tFF\tFF\t77\r\n       345  0CF104A7   00000004    8        F0\t60\t22\tFC\tFF\tFF\tFF\t3B\r\n       344  0CF103A7   00000004    8        17\t1F\t08\t60\tB1\t1F\t08\t3B\r\n       383  0CF101A7   00000004    8        68\t00\t97\tCC\t00\t15\t39\t2D\r\n       382  1FFFFFFF   00000004    8        00\t00\tFF\tFF\tFF\tFF\tFF\tFF\r\n       372  1FFFFFFF   00000004    8        00\t20\tFF\tFF\tFF\tFF\tFF\tFF\r\n       363  0CF102A7   00000004    8        30\t75\tE0\t2E\t80\tFF\tFF\tFD\r\n       363  0CF101A7   00000004    8        68\t00\t97\tCC\t00\t15\t39\t2C\r\n       362  1FFFFFFF   00000004    8        00\t00\tFF\tFF\tFF\tFF\tFF\tFF\r\n       352  1FFFFFFF   00000004    8        00\t00\tFF\tFF\tFF\tFF\tFF\tFF\r\n       347  1FFFFFFF   00000004    8        00\t00\tFF\tFF\tFF\tFF\tFF\tFF\r\n       346  18F121F0   00000004    8        09\t16\t00\t00\tFF\tFF\tB0\t01\r\n       345  18F106A7   00000004    8        00\tF7\tFF\tFF\tFF\tFF\tFF\t77\r\n       345  0CF104A7   00000004    8        F0\t60\t22\tFC\tFF\tFF\tFF\t3B\r\n       383  0CF102A7   00000004    8        30\t75\tE0\t2E\t80\tFF\tFF\tFD\r\n       383  0CF101A7   00000004    8        68\t00\t97\tCC\t00\t15\t39\t2D\r\n       382  1FFFFFFF   00000004    8        00\t00\tFF\tFF\tFF\tFF\tFF\tFF\r\n       372  1FFFFFFF   00000004    8        00\t20\tFF\tFF\tFF\tFF\tFF\tFF\r\n       363  0CF102A7   00000004    8        30\t75\tE0\t2E\t80\tFF\tFF\tFD\r\n       363  0CF101A7   00000004    8        68\t00\t97\tCC\t00\t15\t39\t2C\r\n       362  1FFFFFFF   00000004    8        00\t00\tFF\tFF\tFF\tFF\tFF\tFF\r\n       352  1FFFFFFF   00000004    8        00\t00\tFF\tFF\tFF\tFF\tFF\tFF\r\n       347  1FFFFFFF   00000004    8        00\t00\tFF\tFF\tFF\tFF\tFF\tFF\r\n       346  18F121F0   00000004    8        09\t16\t00\t00\tFF\tFF\tB0\t01\r\n       345  18F106A7   00000004    8        00\tF7\tFF\tFF\tFF\tFF\tFF\t77\r\n       392  1FFFFFFF   00000004    8        00\t00\tFF\tFF\tFF\tFF\tFF\tFF\r\n       383  0CF102A7   00000004    8        30\t75\tE0\t2E\t80\tFF\tFF\tFD\r\n       383  0CF101A7   00000004    8        68\t00\t97\tCC\t00\t15\t39\t2D\r\n       382  1FFFFFFF   00000004    8        00\t00\tFF\tFF\tFF\tFF\tFF\tFF\r\n       372  1FFFFFFF   00000004    8        00\t20\tFF\tFF\tFF\tFF\tFF\tFF\r\n       363  0CF102A7   00000004    8        30\t75\tE0\t2E\t80\tFF\tFF\tFD\r\n       363  0CF101A7   00000004    8        68\t00\t97\tCC\t00\t15\t39\t2C\r\n       362  1FFFFFFF   00000004    8        00\t00\tFF\tFF\tFF\tFF\tFF\tFF\r\n       352  1FFFFFFF   00000004    8        00\t00\tFF\tFF\tFF\tFF\tFF\tFF\r\n       347  1FFFFFFF   00000004    8        00\t00\tFF\tFF\tFF\tFF\tFF\tFF\r\n       346  18F121F0   00000004    8        09\t16\t00\t00\tFF\tFF\tB0\t01\r\n       393  18F106A7   00000004    8        00\tF7\tFF\tFF\tFF\tFF\tFF\t78\r\n       392  1FFFFFFF   00000004    8        00\t00\tFF\tFF\tFF\tFF\tFF\tFF\r\n       383  0CF102A7   00000004    8        30\t75\tE0\t2E\t80\tFF\tFF\tFD\r\n       383  0CF101A7   00000004    8        68\t00\t97\tCC\t00\t15\t39\t2D\r\n       382  1FFFFFFF   00000004    8        00\t00\tFF\tFF\tFF\tFF\tFF\tFF\r\n       372  1FFFFFFF   00000004    8        00\t20\tFF\tFF\tFF\tFF\tFF\tFF\r\n       363  0CF102A7   00000004    8        30\t75\tE0\t2E\t80\tFF\tFF\tFD\r\n       363  0CF101A7   00000004    8        68\t00\t97\tCC\t00\t15\t39\t2C\r\n       362  1FFFFFFF   00000004    8        00\t00\tFF\tFF\tFF\tFF\tFF\tFF\r\n       352  1FFFFFFF   00000004    8        00\t00\tFF\tFF\tFF\tFF\tFF\tFF\r\n       347  1FFFFFFF   00000004    8        00\t00\tFF\tFF\tFF\tFF\tFF\tFF\r\n       402  1FFFFFFF   00000004    8        00\t00\tFF\tFF\tFF\tFF\tFF\tFF\r\n       393  18F106A7   00000004    8        00\tF7\tFF\tFF\tFF\tFF\tFF\t78\r\n       392  1FFFFFFF   00000004    8        00\t00\tFF\tFF\tFF\tFF\tFF\tFF\r\n       383  0CF102A7   00000004    8        30\t75\tE0\t2E\t80\tFF\tFF\tFD\r\n       383  0CF101A7   00000004    8        68\t00\t97\tCC\t00\t15\t39\t2D\r\n       382  1FFFFFFF   00000004    8        00\t00\tFF\tFF\tFF\tFF\tFF\tFF\r\n       372  1FFFFFFF   00000004    8        00\t20\tFF\tFF\tFF\tFF\tFF\tFF\r\n       363  0CF102A7   00000004    8        30\t75\tE0\t2E\t80\tFF\tFF\tFD\r\n       363  0CF101A7   00000004    8        68\t00\t97\tCC\t00\t15\t39\t2C\r\n       362  1FFFFFFF   00000004    8        00\t00\tFF\tFF\tFF\tFF\tFF\tFF\r\n       352  1FFFFFFF   00000004    8        00\t00\tFF\tFF\tFF\tFF\tFF\tFF\r\n       403  0CF101A7   00000004    8        68\t00\t97\tCC\t00\t15\t39\t2E\r\n       402  1FFFFFFF   00000004    8        00\t00\tFF\tFF\tFF\tFF\tFF\tFF\r\n       393  18F106A7   00000004    8        00\tF7\tFF\tFF\tFF\tFF\tFF\t78\r\n       392  1FFFFFFF   00000004    8        00\t00\tFF\tFF\tFF\tFF\tFF\tFF\r\n       383  0CF102A7   00000004    8        30\t75\tE0\t2E\t80\tFF\tFF\tFD\r\n       383  0CF101A7   00000004    8        68\t00\t97\tCC\t00\t15\t39\t2D\r\n       382  1FFFFFFF   00000004    8        00\t00\tFF\tFF\tFF\tFF\tFF\tFF\r\n       372  1FFFFFFF   00000004    8        00\t20\tFF\tFF\tFF\tFF\tFF\tFF\r\n       363  0CF102A7   00000004    8        30\t75\tE0\t2E\t80\tFF\tFF\tFD\r\n       363  0CF101A7   00000004    8        68\t00\t97\tCC\t00\t15\t39\t2C\r\n       362  1FFFFFFF   00000004    8        00\t00\tFF\tFF\tFF\tFF\tFF\tFF\r\n       403  0CF102A7   00000004    8        30\t75\tE0\t2E\t80\tFF\tFF\tFD\r\n       403  0CF101A7   00000004    8        68\t00\t97\tCC\t00\t15\t39\t2E\r\n       402  1FFFFFFF   00000004    8        00\t00\tFF\tFF\tFF\tFF\tFF\tFF\r\n       393  18F106A7   00000004    8        00\tF7\tFF\tFF\tFF\tFF\tFF\t78\r\n       392  1FFFFFFF   00000004    8        00\t00\tFF\tFF\tFF\tFF\tFF\tFF\r\n       383  0CF102A7   00000004    8        30\t75\tE0\t2E\t80\tFF\tFF\tFD\r\n       383  0CF101A7   00000004    8        68\t00\t97\tCC\t00\t15\t39\t2D\r\n       382  1FFFFFFF   00000004    8        00\t00\tFF\tFF\tFF\tFF\tFF\tFF\r\n       372  1FFFFFFF   00000004    8        00\t20\tFF\tFF\tFF\tFF\tFF\tFF\r\n       363  0CF102A7   00000004    8        30\t75\tE0\t2E\t80\tFF\tFF\tFD\r\n       363  0CF101A7   00000004    8        68\t00\t97\tCC\t00\t15\t39\t2C\r\n       412  1FFFFFFF   00000004    8        00\t20\tFF\tFF\tFF\tFF\tFF\tFF\r\n       403  0CF102A7   00000004    8        30\t75\tE0\t2E\t80\tFF\tFF\tFD\r\n       403  0CF101A7   00000004    8        68\t00\t97\tCC\t00\t15\t39\t2E\r\n       402  1FFFFFFF   00000004    8        00\t00\tFF\tFF\tFF\tFF\tFF\tFF\r\n       393  18F106A7   00000004    8        00\tF7\tFF\tFF\tFF\tFF\tFF\t78\r\n       392  1FFFFFFF   00000004    8        00\t00\tFF\tFF\tFF\tFF\tFF\tFF\r\n       383  0CF102A7   00000004    8        30\t75\tE0\t2E\t80\tFF\tFF\tFD\r\n       383  0CF101A7   00000004    8        68\t00\t97\tCC\t00\t15\t39\t2D\r\n       382  1FFFFFFF   00000004    8        00\t00\tFF\tFF\tFF\tFF\tFF\tFF\r\n       372  1FFFFFFF   00000004    8        00\t20\tFF\tFF\tFF\tFF\tFF\tFF\r\n       363  0CF102A7   00000004    8        30\t75\tE0\t2E\t80\tFF\tFF\tFD\r\n       422  1FFFFFFF   00000004    8        00\t00\tFF\tFF\tFF\tFF\tFF\tFF\r\n       412  1FFFFFFF   00000004    8        00\t20\tFF\tFF\tFF\tFF\tFF\tFF\r\n       403  0CF102A7   00000004    8        30\t75\tE0\t2E\t80\tFF\tFF\tFD\r\n       403  0CF101A7   00000004    8        68\t00\t97\tCC\t00\t15\t39\t2E\r\n       402  1FFFFFFF   00000004    8        00\t00\tFF\tFF\tFF\tFF\tFF\tFF\r\n       393  18F106A7   00000004    8        00\tF7\tFF\tFF\tFF\tFF\tFF\t78\r\n       392  1FFFFFFF   00000004    8        00\t00\tFF\tFF\tFF\tFF\tFF\tFF\r\n       383  0CF102A7   00000004    8        30\t75\tE0\t2E\t80\tFF\tFF\tFD\r\n       383  0CF101A7   00000004    8        68\t00\t97\tCC\t00\t15\t39\t2D\r\n       382  1FFFFFFF   00000004    8        00\t00\tFF\tFF\tFF\tFF\tFF\tFF\r\n       372  1FFFFFFF   00000004    8        00\t20\tFF\tFF\tFF\tFF\tFF\tFF\r\n       423  0CF101A7   00000004    8        68\t00\t97\tCC\t00\t15\t39\t2F\r\n       422  1FFFFFFF   00000004    8        00\t00\tFF\tFF\tFF\tFF\tFF\tFF\r\n       412  1FFFFFFF   00000004    8        00\t20\tFF\tFF\tFF\tFF\tFF\tFF\r\n       403  0CF102A7   00000004    8        30\t75\tE0\t2E\t80\tFF\tFF\tFD\r\n       403  0CF101A7   00000004    8        68\t00\t97\tCC\t00\t15\t39\t2E\r\n       402  1FFFFFFF   00000004    8        00\t00\tFF\tFF\tFF\tFF\tFF\tFF\r\n       393  18F106A7   00000004    8        00\tF7\tFF\tFF\tFF\tFF\tFF\t78\r\n       392  1FFFFFFF   00000004    8        00\t00\tFF\tFF\tFF\tFF\tFF\tFF\r\n       383  0CF102A7   00000004    8        30\t75\tE0\t2E\t80\tFF\tFF\tFD\r\n       383  0CF101A7   00000004    8        68\t00\t97\tCC\t00\t15\t39\t2D\r\n       382  1FFFFFFF   00000004    8        00\t00\tFF\tFF\tFF\tFF\tFF\tFF\r\n       423  0CF102A7   00000004    8        30\t75\tE0\t2E\t80\tFF\tFF\tFD\r\n       423  0CF101A7   00000004    8        68\t00\t97\tCC\t00\t15\t39\t2F\r\n       422  1FFFFFFF   00000004    8        00\t00\tFF\tFF\tFF\tFF\tFF\tFF\r\n       412  1FFFFFFF   00000004    8        00\t20\tFF\tFF\tFF\tFF\tFF\tFF\r\n       403  0CF102A7   00000004    8        30\t75\tE0\t2E\t80\tFF\tFF\tFD\r\n       403  0CF101A7   00000004    8        68\t00\t97\tCC\t00\t15\t39\t2E\r\n       402  1FFFFFFF   00000004    8        00\t00\tFF\tFF\tFF\tFF\tFF\tFF\r\n       393  18F106A7   00000004    8        00\tF7\tFF\tFF\tFF\tFF\tFF\t78\r\n       392  1FFFFFFF   00000004    8        00\t00\tFF\tFF\tFF\tFF\tFF\tFF\r\n       383  0CF102A7   00000004    8        30\t75\tE0\t2E\t80\tFF\tFF\tFD\r\n       383  0CF101A7   00000004    8        68\t00\t97\tCC\t00\t15\t39\t2D\r\n       432  1FFFFFFF   00000004    8        00\t00\tFF\tFF\tFF\tFF\tFF\tFF\r\n       423  0CF102A7   00000004    8        30\t75\tE0\t2E\t80\tFF\tFF\tFD\r\n       423  0CF101A7   00000004    8        68\t00\t97\tCC\t00\t15\t39\t2F\r\n       422  1FFFFFFF   00000004    8        00\t00\tFF\tFF\tFF\tFF\tFF\tFF\r\n       412  1FFFFFFF   00000004    8        00\t20\tFF\tFF\tFF\tFF\tFF\tFF\r\n       403  0CF102A7   00000004    8        30\t75\tE0\t2E\t80
